vi "FIFO Core U64 - SRAM.vi"(0 "input data":u64, 1 "reset":bool, 2 "resources":T1={"io resources"={"address"="SRAM\\Address", "command"="SRAM\\Command", "push_fifo"="SRAM\\Push_Fifo", "write_data"="SRAM\\Write_Data", "read_data"="SRAM\\Read_Data", "read_data_valid"="SRAM\\Read_Data_Valid", "fifo_full"="SRAM\\Fifo_Full"}}, 3 "fifo depth":u8(ring)=10 items=["4"=2, "8"=3, "16"=4, "32"=5, "64"=6, "128"=7, "256"=8, "512"=9, "1024"=10, "2048"=11, "4096"=12, "8192"=13, "16384"=14, "32768"=15, "65536"=16, "131072"=17, "262144"=18, "524288"=19, "1048576"=20, "2097152"=21, "4194304"=22, "8388608"=23, "16777216"=24, "33554432"=25, "67108864"=26, "134217728"=27, "268435456"=28, "536870912"=29, "1073741824"=30, "2147483648"=31, "4294967296"=32], 9 "input valid":bool, 12 "ready for output":bool=TRUE) -> (4 "output data":u64, 6 "state":T2, 10 "output valid":bool, 14 "ready for input":bool)   [LabVIEW 2011, in "FIFO.lvlib"]
uses:
  <instrlib>/RF-RIO/FIFO/FIFO/FPGA/FIFO.lvlib
  <instrlib>/RF-RIO/FIFO/FIFO/FPGA/Public/FIFO State.ctl
  <instrlib>/FlexRIO/Libraries/Memory/FPGA/Interface/Read Request.ctl
  <instrlib>/RF-RIO/Memory/1.0.0/FPGA/Public/Write Data (64-Bit No Byte Enables).ctl
  <instrlib>/RF-RIO/Memory/1.0.0/FPGA/Private/Process (SRAM 64-Bit).vi
  <instrlib>/FlexRIO/Libraries/Memory/FPGA/Memory.lvlib
  <instrlib>/RF-RIO/Memory/1.0.0/FPGA/niRFRIO Memory 1.0.0 FPGA.lvlib
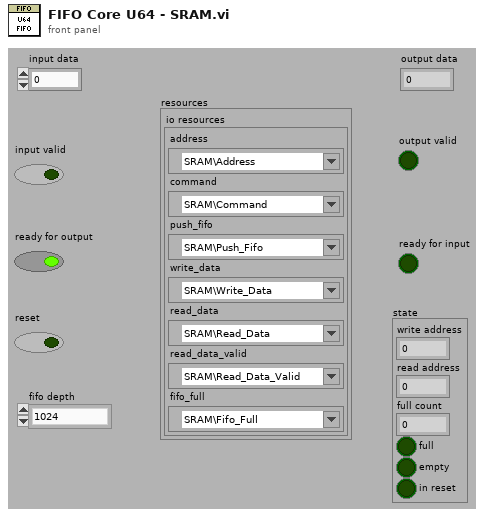
[diagram p1: front panel]
types:
  T1 = cluster{"io resources":cluster{"address":refnum<k21>, "command":refnum<k21>, "push_fifo":refnum<k21>, "write_data":refnum<k21>, "read_data":refnum<k21>, "read_data_valid":refnum<k21>, "fifo_full":refnum<k21>}}
  T2 = typedef "FIFO.lvlib/FIFO State.ctl" = cluster{"write address":u32, "read address":u32, "full count":u32, "full":bool, "empty":bool, "in reset":bool}
  T3 = typedef "FIFO.lvlib/niRFRIO Memory 1.0.0 FPGA.lvlib/Write Data (64-Bit No Byte Enables).ctl" = cluster{"address":u32, "data":u64, "valid":bool}
  T4 = typedef "Memory.lvlib/Read Request.ctl" = cluster{"address":u32, "valid":bool}
  T5 = typedef "FIFO.lvlib/FIFO State - 32-bit Address.ctl" = cluster{"write address":u32, "read address":u32, "full count":u32, "full":bool, "empty":bool}
  T6 = typedef "FIFO.lvlib/niRFRIO Memory 1.0.0 FPGA.lvlib/Retrieve Data (64-Bit).ctl" = cluster{"data":u64, "valid":bool}
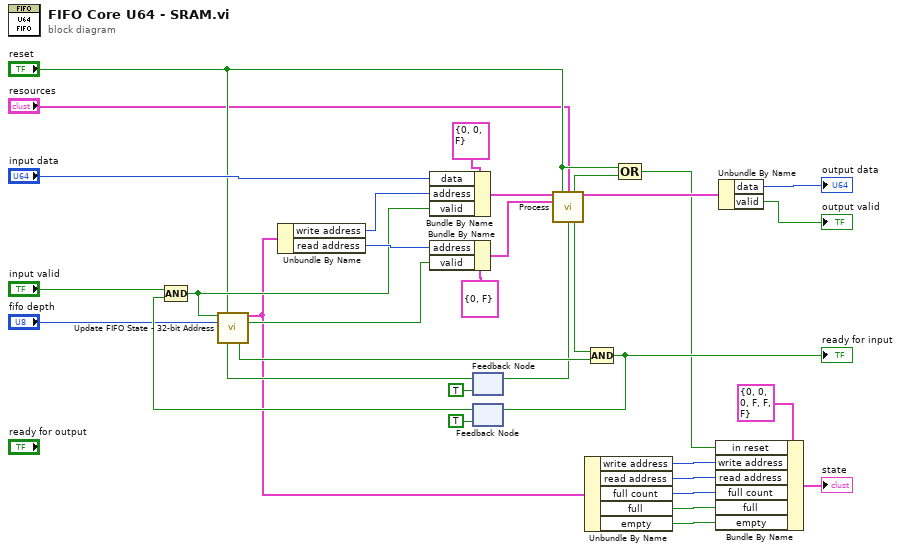
[diagram p0: block diagram]
diagram:
  n1 = feedback #1(TRUE ("ready for read request")) -> (w21:bool)
  n2 = feedback #2(TRUE) -> (w25:bool)
  n3 = Compound Arithmetic op=AND("input valid", w25) -> (w19:bool)
  n4 = call <instrlib>:"Update FIFO State - 32-bit Address.vi"("issue write"=w19, "reset"="reset", "fifo depth"="fifo depth", "ready for read request"=w21) -> ("state"=w8:T5, "issue read request"=w22:bool, "ready for write"=w24:bool)  [unwired: 9 in]
  n5 = Unbundle By Name(w8) -> ("write address"=w33:u32, "read address"=w31:u32)
  n6 = Bundle By Name(cluster=T3 {"address"=0, "data"=0, "valid"=FALSE} ("write data"), "data"="input data", "address"=w33, "valid"=w19) -> (w2:T3)
  n7 = Bundle By Name(cluster=T4 {"address"=0, "valid"=FALSE} ("read request"), "address"=w31, "valid"=w22) -> (w4:T4)
  n8 = call-poly <instrlib>:"Process.vi"("write data"=w2, "reset"="reset", "resources"="resources", "read request"=w4) -> ("in reset"=w11:bool, "retrieve data"=w29:T6, "ready for read request"=w23:bool, "ready for write"=w1:bool)  [unwired: 8 in]
  n9 = feedback-in #1(w23) -> ()
  n10 = Unbundle By Name(w8) -> ("write address"=w17:u32, "read address"=w16:u32, "full count"=w15:u32, "full"=w14:bool, "empty"=w13:bool)
  n11 = Compound Arithmetic op=AND(w1, w24) -> (w26:bool)
  "ready for input" <- w26
  n12 = feedback-in #2(w26) -> ()
  n13 = Compound Arithmetic op=OR("reset", w11) -> (w9:bool)
  n14 = Bundle By Name(cluster=T2 {"write address"=0, "read address"=0, "full count"=0, "full"=FALSE, "empty"=FALSE, "in reset"=FALSE} ("state"), "in reset"=w9, "write address"=w17, "read address"=w16, "full count"=w15, "full"=w14, "empty"=w13) -> (→"state":T2)
  n15 = Unbundle By Name(w29) -> ("data"=→"output data":u64, "valid"=→"output valid":bool)
